vi "GlobalImage.vi"() -> ()   [LabVIEW 2013]
panel:
  out "CurrentImage":dbl[][](array[numeric])
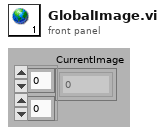
[diagram p1: front panel]
diagram:
